vi "Pololu.Mgr - Get Device Config for Channel.vi"(10 "Channel":u8, 11 "Devices":T1[](array[typedef])) -> (2 "Device":T1, 3 "Devices Out":T1[](array[typedef]), 5 "Index":i32)   [LabVIEW 2018]
uses:
  SubVIs/Pololu.Device Config.ctl
  SubVIs/Pololu.Device Range Config.ctl
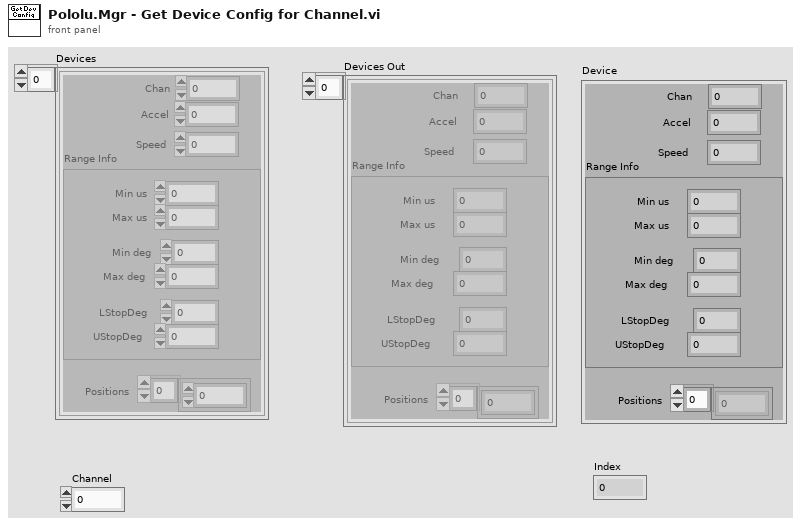
[diagram p1: front panel]
types:
  T1 = typedef "Pololu.Device Config.ctl" = cluster{"Chan":u8, "Accel":u16, "Speed":u16, "Positions":dbl[], "Range Info":T2}
  T2 = typedef "Pololu.Device Range Config.ctl" = cluster{"Min us":dbl, "Max us":dbl, "Min deg":dbl, "Max deg":dbl, "LStopDeg":dbl, "UStopDeg":dbl}
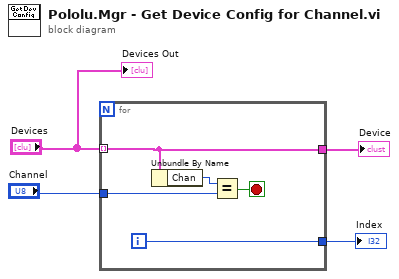
[diagram p0: block diagram]
diagram:
  n1 = for {
    tunnel: "Devices" -> [w8] mode=indexing
    tunnel: [w9] -> w4
    tunnel: [w8] -> w2
    tunnel: "Channel" -> [w6]
    i -> [w9]
    stop <- w5 stop-if-true
    n2 = Unbundle By Name(w8) -> ("Chan"=w7:u8)
    n3 = Equal?(x=w7, y=w6) -> (x = y?=w5:bool)
  }
  "Index" <- w4
  "Device" <- w2
  "Devices Out" <- "Devices"
